vi "Valves Global.vi"(8 "Action":T2, 9 "Valve States":bool[](array[boolean]), 10 "Valve Buttons":refnum<vi>[](array[refnum]), 11 "Valves":T1[](array[typedef])=[enum."SOL0", enum."COMP", enum."COMP", enum."SOL0", enum."SOL0", enum."COMP", enum."COMP"]) -> (0 "Valve Update Occurrence":refnum<k4>, 1 "States":bool[](array[boolean]), 2 "Buttons":refnum<vi>[](array[refnum]), 3 "Valves":T1[](array[typedef]))   [LabVIEW 2015]
uses:
  Valve Button Mapping Global Action.ctl
  Valve Name Enum.ctl
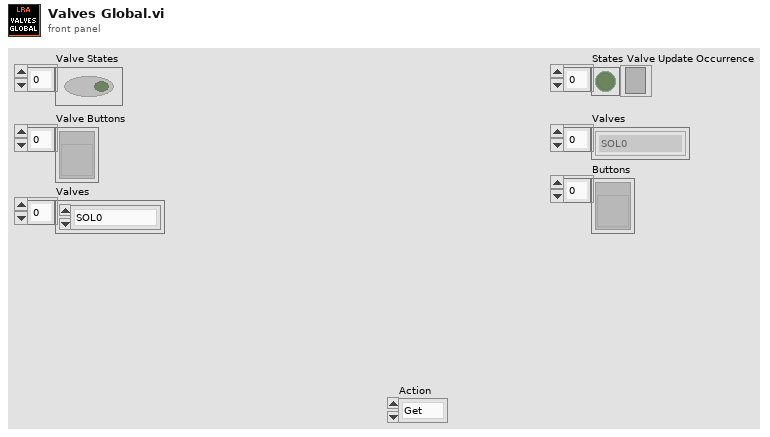
[diagram p1: front panel]
types:
  T1 = typedef "Valve Name Enum.ctl" = enum16{"SOL0", "COMP"}
  T2 = typedef "Valve Button Mapping Global Action.ctl" = enum16{"Get", "Set", "Init"}
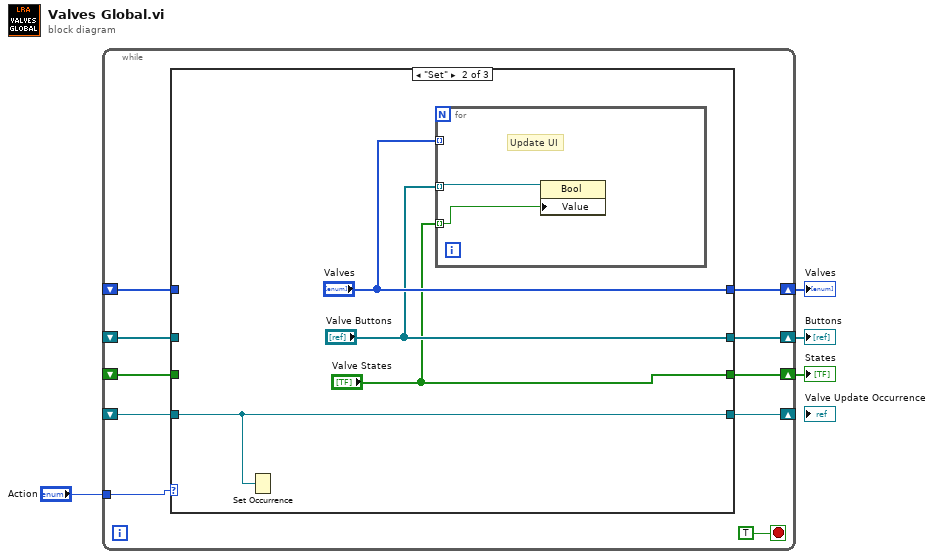
[diagram p0: block diagram]
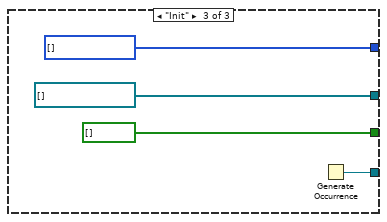
[diagram p3: hidden frame]
diagram:
  n1 = while {
    tunnel: "Action" -> [w13]
    shift-right: [w12] -> w3
    shift-left: _ -> [w10]
    shift-right: [w11] -> w2
    shift-left: _ -> [w9]
    shift-right: [w7] -> w1
    shift-left: _ -> [w8]
    shift-right: [w6] -> _
    shift-left: _ -> [w5]
    stop <- TRUE stop-if-true
    n2 = case shown="\"Set\"" w13 {
      tunnel: [w18 "Valves" w28] -> w12
      tunnel: [w17 "Valve Buttons" refnum<vi>[] [] ("Valve Buttons")] -> w11
      tunnel: w10 -> [w18 _ _]
      tunnel: w9 -> [w17 _ _]
      tunnel: w8 -> [w16 _ _]
      tunnel: [w16 "Valve States" bool[] [] ("Valve States")] -> w7
      tunnel: [w15 w22 w25] -> w6
      tunnel: w5 -> [w15 w22 _]
      frame "Get", Default {
      }
      frame "Set" {
        n3 = Set Occurrence(w22) -> ()
        n4 = for {
          tunnel: "Valves" -> [_] mode=indexing
          tunnel: "Valve Buttons" -> [w24] mode=indexing
          tunnel: "Valve States" -> [w23] mode=indexing
          # "Update UI"
          n5 = property class="Bool"(reference=w24, "Value"=w23) -> ()  [unwired: 1 in, 2 out]
        }
      }
      frame "Init" {
        w28 = T1[] [] items=["SOL0", "COMP"] ("Valves")
        n6 = Generate Occurrence() -> (w25:refnum<k4>)
      }
    }
  }
  "Valves" <- w3
  "Buttons" <- w2
  "States" <- w1
